vi "Read Visible.vi"(9 "Decoration in":refnum<class "Decoration.lvclass">) -> (3 "Decoration out":refnum<class "Decoration.lvclass">, 4 "Visible":bool)   [LabVIEW 2014, in "Decoration.lvclass"]
uses:
  Decoration.lvclass
  Decoration.lvclass/Decoration.ctl
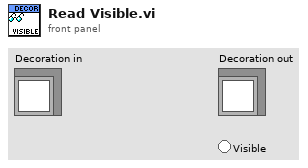
[diagram p1: front panel]
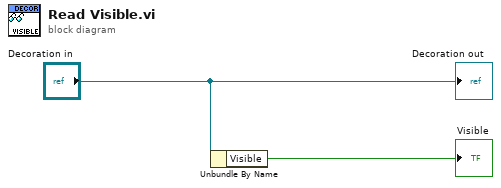
[diagram p0: block diagram]
diagram:
  n1 = Unbundle By Name("Decoration in") -> ("Visible"=→"Visible":bool)
  "Decoration out" <- "Decoration in"
